vi "TestIOInit.vi"(4 "ConfigData":string, 5 "IODeviceName":string) -> (0 "Parameter OK":bool, 1 "IOData":T1, 2 "VI Refnum":refnum<vi>)   [LabVIEW 2020]
uses:
  <vilib>/Utility/error.llb/DialogType.ctl
panel:
  in  "InPorts":i32
  in  "OutPorts":i32
  in  "InStart":string
  in  "OutStart":string
  in  "ID":string
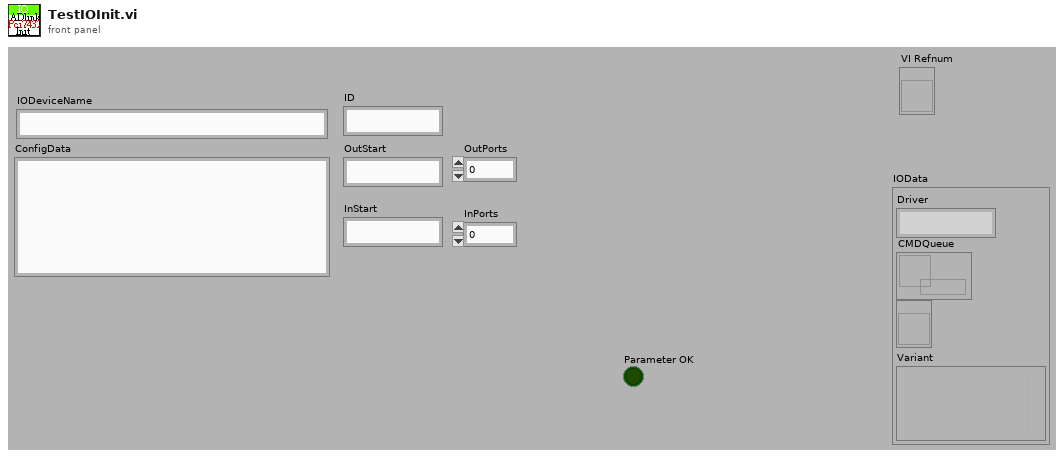
[diagram p1: front panel]
types:
  T1 = cluster{"Driver":string, "CMDQueue":refnum<queue>, refnum<vi>, "Variant":variant}
  T2 = cluster{"Command":string, "Parameter":string, "queue out":refnum<queue>}
  T3 = typedef "DialogType.ctl" = u16
  T4 = cluster{"Variant":variant, "trimmed string":string, "ID":string, "OutStart":string, "OutPorts":i32, "InStart":string, "InPorts":i32}
  T5 = cluster{"Driver":string, "queue out":refnum<queue>, refnum<vi>, "Variant":variant}
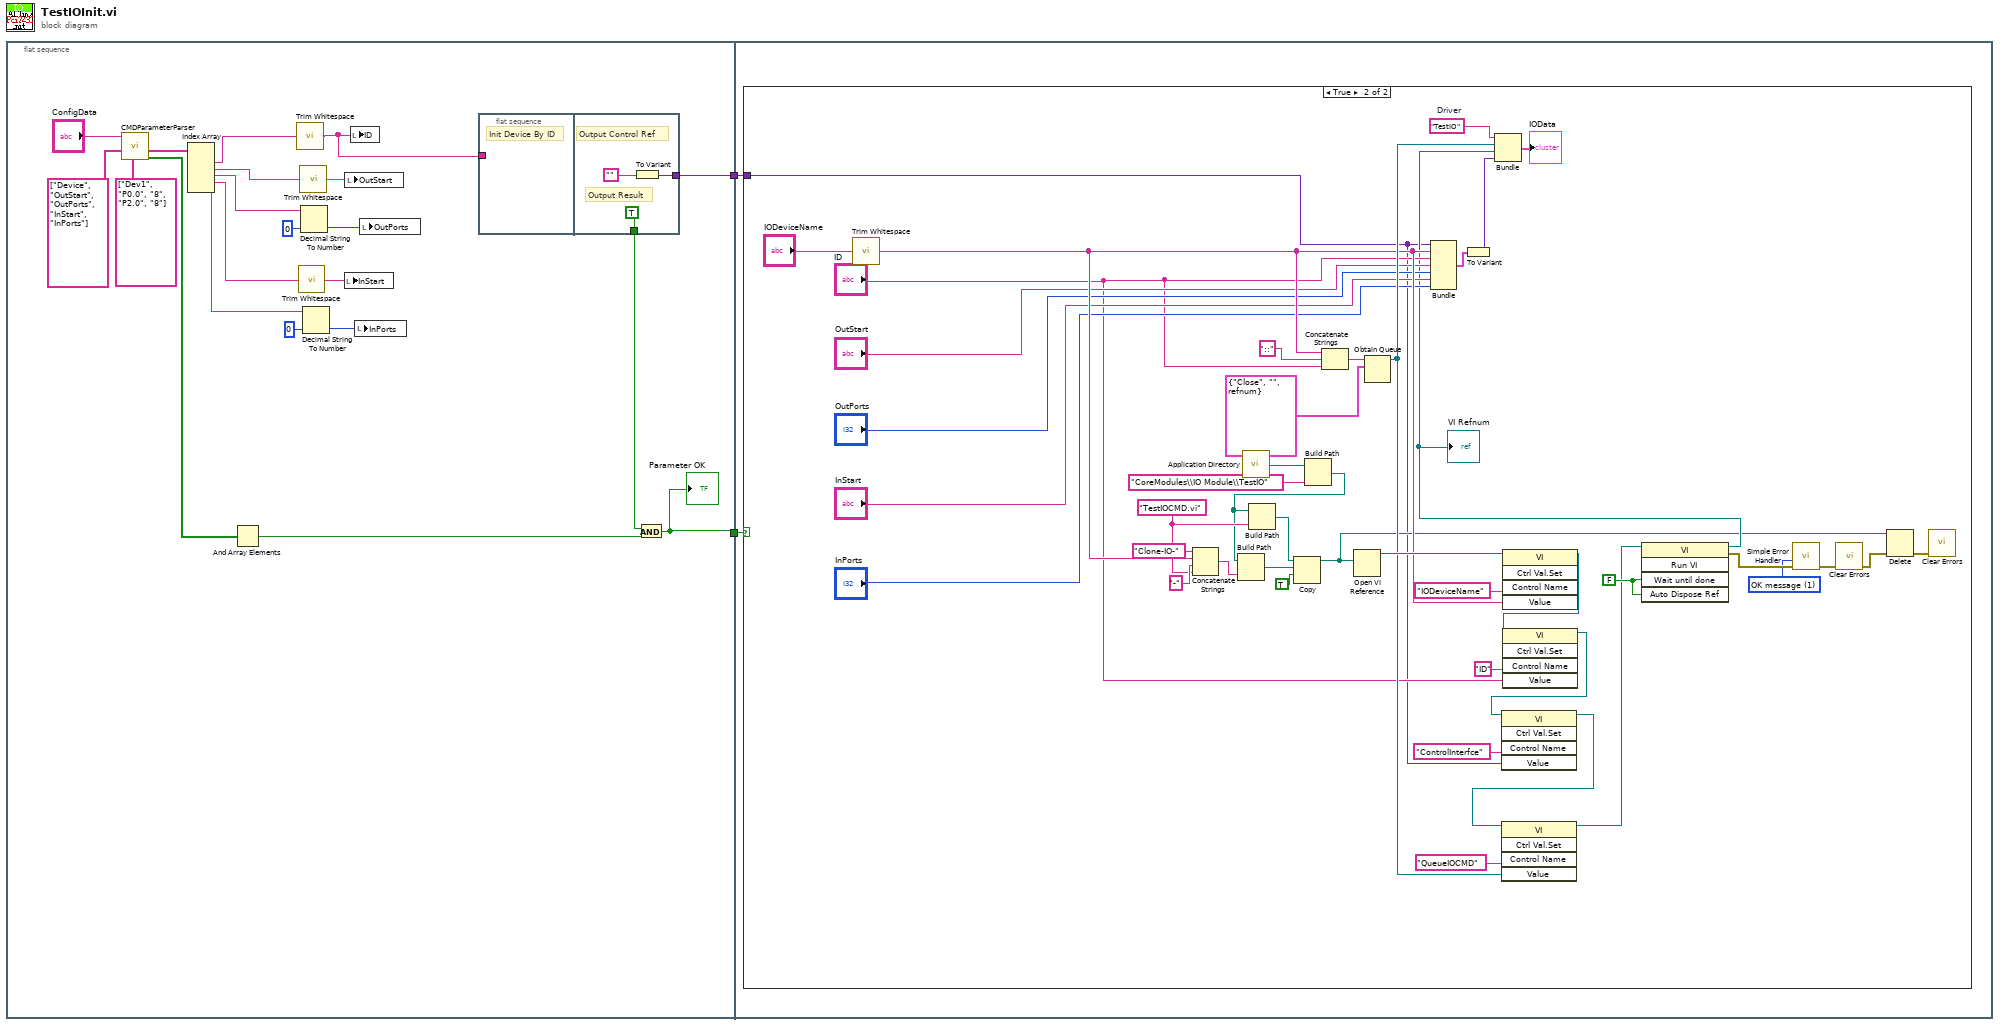
[diagram p0: block diagram]
diagram:
  n1 = flat-sequence {
    tunnel: [w23] -> w2
    tunnel: [w16] -> w1
    tunnel: w2 -> [w28]
    tunnel: w1 -> [w27]
    frame #0 {
      n2 = call "CMDParameterParser.vi"("DeafultValues"=string[] ["Dev1", "P0.0", "8", "P2.0", "8"] ("ParameterKey"), "RequiredKeys"=string[] ["Device", "OutStart", "OutPorts", "InStart", "InPorts"] ("ParameterKey"), "CMDParameter"="ConfigData") -> ("KeyFind?"=w4:bool[], "KeyValues"=w12:string[])  [unwired: 6 in, 1 out]
      n3 = Index Array(array=w12) -> (element #1=w11:string, element #2=w10:string, element #3=w9:string, element #4=w8:string, element #5=w7:string)  [unwired: 5 in]
      n4 = And Array Elements(Boolean array=w4) -> (logical AND=w3:bool)
      n5 = call <vilib>:"Trim Whitespace.vi"("string"=w11) -> ("trimmed string"=w6:string)  [unwired: 1 in]
      n6 = call <vilib>:"Trim Whitespace.vi"("string"=w8) -> ("trimmed string"=w17:string)  [unwired: 1 in]
      n7 = call <vilib>:"Trim Whitespace.vi"("string"=w10) -> ("trimmed string"=w18:string)  [unwired: 1 in]
      n8 = Decimal String To Number(string=w9, default (0L)=0 ("default (0 I32)")) -> (number=w21:i32)  [unwired: 1 in, 1 out]
      n9 = Decimal String To Number(string=w7, default (0L)=0 ("default (0 I32)")) -> (number=w19:i32)  [unwired: 1 in, 1 out]
      n10 = local write "InStart"(w17) -> ()
      n11 = local write "OutStart"(w18) -> ()
      n12 = local write "ID"(w6) -> ()
      n13 = local write "InPorts"(w19) -> ()
      n14 = local write "OutPorts"(w21) -> ()
      n15 = flat-sequence {
        tunnel: w6 -> [_]
        tunnel: [w24] -> w16
        tunnel: [TRUE ("x")] -> w5
        frame #0 {
          # "Init Device By ID"
        }
        frame #1 {
          # "Output Result"
          # "Output Control Ref"
          n16 = To Variant(anything="") -> (Variant=w24:variant)
        }
      }
      n17 = And(x=w5, y=w3) -> (x .and. y?=w23:bool)
      "Parameter OK" <- w23
    }
    frame #1 {
      n18 = case shown="True" w28 {
        tunnel: w27 -> [_ w35]
        frame False {
        }
        frame True {
          w33 = T3 1 items=["no dialog", "OK message", "continue or stop message", "OK message + warnings", "continue/stop + warnings"] ("type of dialog (OK msg:1)")
          w51 = FALSE ("Wait Until Done")
          w62 = "TestIOCMD.vi" ("name or relative path")
          w67 = "TestIO"  # Driver
          n19 = call <vilib>:"Trim Whitespace.vi"("string"="IODeviceName") -> ("trimmed string"=w49:string)  [unwired: 1 in]
          n20 = Concatenate Strings("Clone-IO-" ("string"), w49, "-" ("string"), w62) -> (w66:string)
          n21 = call <vilib>:"Application Directory.vi"() -> ("Application Directory"=w39:path)
          n22 = Build Path(base path=w39, name or relative path="CoreModules\\IO Module\\TestIO") -> (appended path=w37:path)
          n23 = Build Path(base path=w37, name or relative path=w66) -> (appended path=w64:path)
          n24 = Build Path(base path=w37, name or relative path=w62) -> (appended path=w61:path)
          n25 = Copy(9:TRUE ("overwrite (F)"), 10:w64, 11:w61) -> (3:w36:path)  [unwired: 2 in, 2 out]
          n26 = Concatenate Strings(w49, "::" ("string"), "ID") -> (w70:string)
          n27 = Open VI Reference(vi path=w36) -> (vi reference=w56:refnum<vi>)  [unwired: 5 in, 1 out]
          n28 = Obtain Queue(name (unnamed)=w70, element data type=T2 {"Command"="Close", "Parameter"="", "queue out"=refnum} ("Motor Module CMD")) -> (queue out=w55:refnum<queue>)  [unwired: 3 in, 2 out]
          n29 = Bundle("Variant"=w35, "trimmed string"=w49, "ID"="ID", "OutStart"="OutStart", "OutPorts"="OutPorts", "InStart"="InStart", "InPorts"="InPorts") -> (w71:T4)  [unwired: 1 in]
          n30 = To Variant(anything=w71) -> (Variant=w42:variant)
          n31 = invoke class="VI" method="Ctrl Val.Set"(reference=w56, "Control Name"="IODeviceName", "Value"=w49) -> (reference out=w54:refnum<vi>)  [unwired: 2 in, 4 out]
          n32 = invoke class="VI" method="Ctrl Val.Set"(reference=w54, "Control Name"="ID", "Value"="ID") -> (reference out=w53:refnum<vi>)  [unwired: 2 in, 4 out]
          n33 = invoke class="VI" method="Ctrl Val.Set"(reference=w53, "Control Name"="ControlInterfce", "Value"=w35) -> (reference out=w52:refnum<vi>)  [unwired: 2 in, 4 out]
          n34 = invoke class="VI" method="Ctrl Val.Set"(reference=w52, "Control Name"="QueueIOCMD", "Value"=w55) -> (reference out=w29:refnum<vi>)  [unwired: 2 in, 4 out]
          n35 = invoke class="VI" method="Run VI"(reference=w29, "Wait until done"=w51, "Auto Dispose Ref"=w51) -> (reference out=w41:refnum<vi>, error out=w34:errorcluster)  [unwired: 2 in, 3 out]
          "VI Refnum" <- w41
          n36 = Bundle("Driver"=w67, "queue out"=w55, w41, "Variant"=w42) -> (→"IOData":T5)  [unwired: 1 in]
          n37 = call <vilib>:"Simple Error Handler.vi"("type of dialog (OK msg:1)"=w33, "error in (no error)"=w34) -> ("error out"=w32:errorcluster)  [unwired: 3 in, 4 out]
          n38 = call <vilib>:"Clear Errors.vi"("error in (no error)"=w32) -> ("error out"=w31:errorcluster)  [unwired: 5 in, 1 out]
          n39 = Delete(path (use dialog)=w36, error in=w31) -> (error out=w30:errorcluster)  [unwired: 3 in, 2 out]
          n40 = call <vilib>:"Clear Errors.vi"("error in (no error)"=w30) -> ()  [unwired: 5 in, 2 out]
        }
      }
    }
  }
